vi "build event cluster start.vi"(0 "position in [km]":sgl, 11 "time cluster in":T1) -> (8 "event data out":T2)   [LabVIEW 2014]
uses:
  typedefs/event cluster typedef.ctl
  typedefs/time cluster typedef.ctl
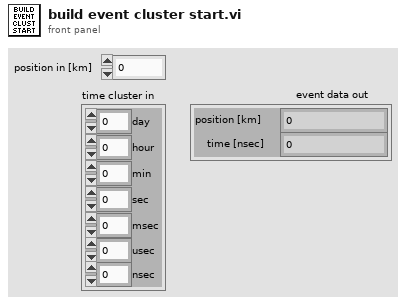
[diagram p1: front panel]
types:
  T1 = typedef "time cluster typedef.ctl" = cluster{"day":u32, "hour":u32, "min":u32, "sec":u32, "msec":u32, "usec":u32, "nsec":u32}
  T2 = typedef "event cluster typedef.ctl" = cluster{"position [km]":sgl, "time [nsec]":i64}
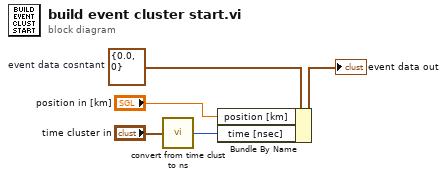
[diagram p0: block diagram]
diagram:
  w3 = T2 {"position [km]"=0.0, "time [nsec]"=0}  # event data cosntant
  n1 = call "convert from time clust to ns.vi"("time cluster"="time cluster in") -> ("time (nsec)"=w2:i64)  [unwired: 14 in]
  n2 = Bundle By Name(cluster=w3, "position [km]"="position in [km]", "time [nsec]"=w2) -> (→"event data out":T2)
